vi "EnFlo_Error_Handler.vi"(3 "error in (no error)":errorcluster, 4 "Error Type":string, 5 "Dialog Box (T)":bool=TRUE) -> (0 "Continue":bool, 1 "SMS Message":string, 2 "Email Message":string)   [LabVIEW 2016]
uses:
  Controls/Post_Process.ctl
  <vilib>/Utility/error.llb/DialogType.ctl
  Globals/Meas_global.vi
  Globals/Trav_pos_global.vi
  Globals/Preference_global.vi
  Email_transfer_global.vi
  Globals/Dynamic_call_global.ph.vi
panel:
  out "error out":errorcluster
  in  "Case Constant\n(See Context Help)":bool
  out "Server copy Location":path
  out "Hours Running":dbl format="%.2f"
  out "Error Information":string
  out "Log Files":path[](array[path])
  out "Frequency":i32
  out "Error Analysis":string
  out "Error Types":string[](array[string])
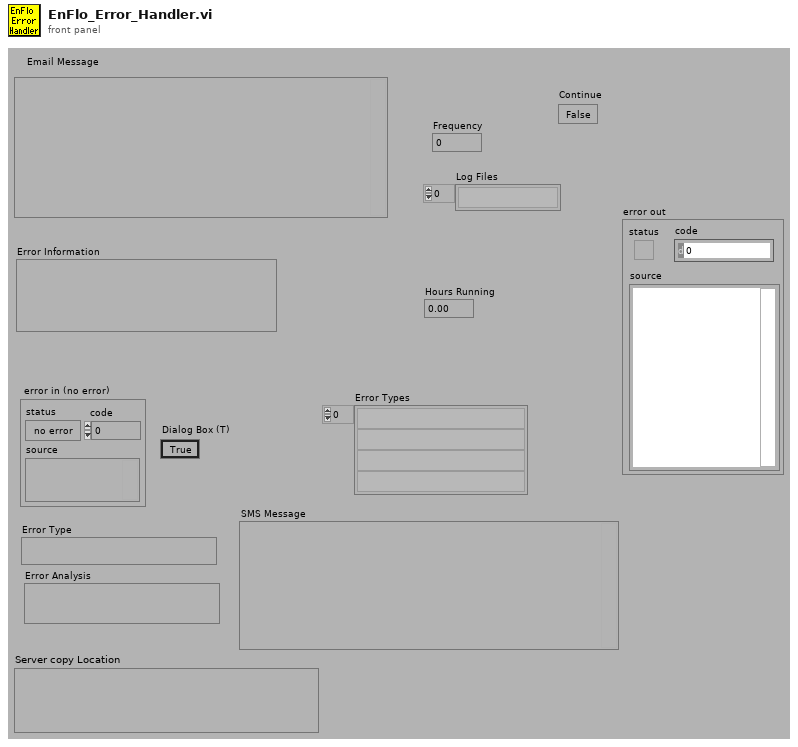
[diagram p1: front panel]
types:
  T1 = typedef "Post_Process.ctl" = enum16{"Take New Data", "Post Process Raw Data File"}
  T2 = cluster{"path":path, "data":string, "binary":bool, "MIME content-type \n(application/octet-stream)":string}[]
  T3 = typedef "DialogType.ctl" = u16
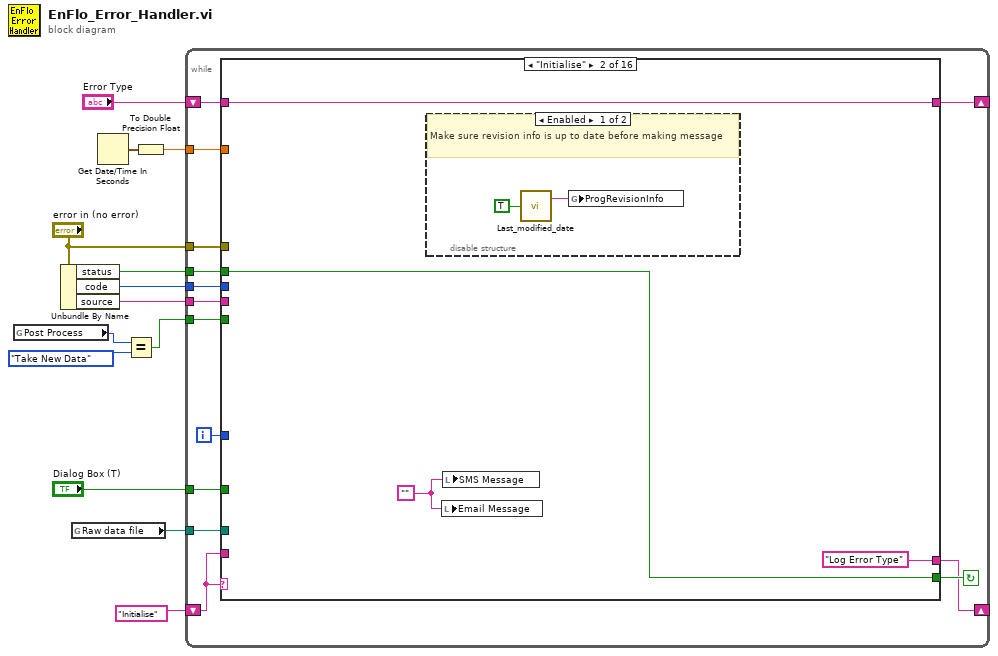
[diagram p0: block diagram]
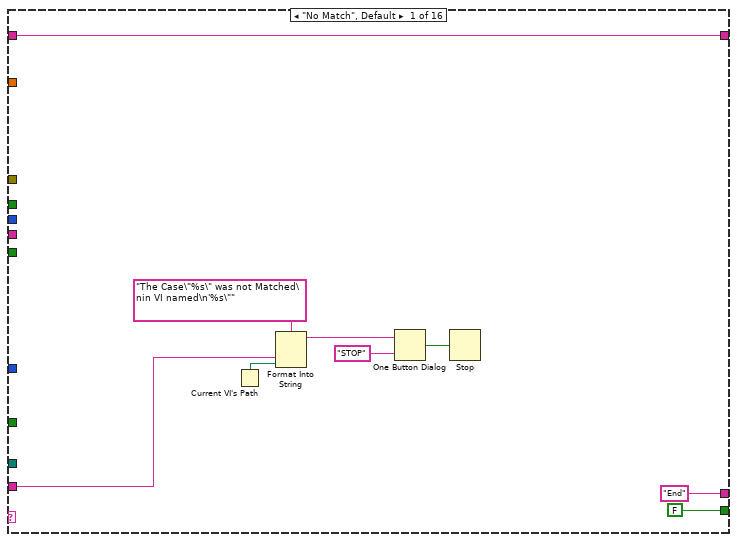
[diagram p2: hidden frame]
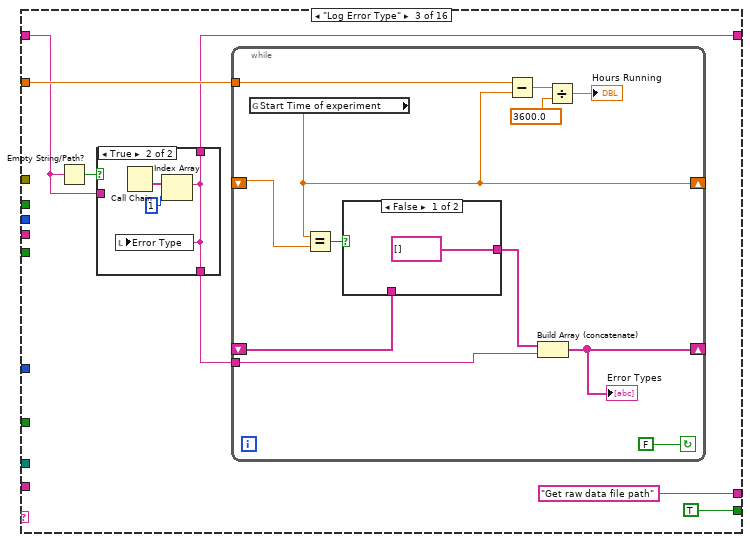
[diagram p4: hidden frame]
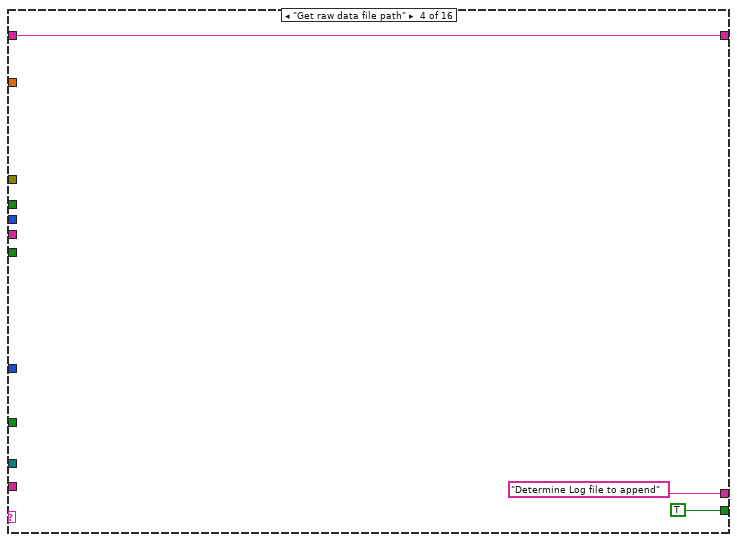
[diagram p7: hidden frame]
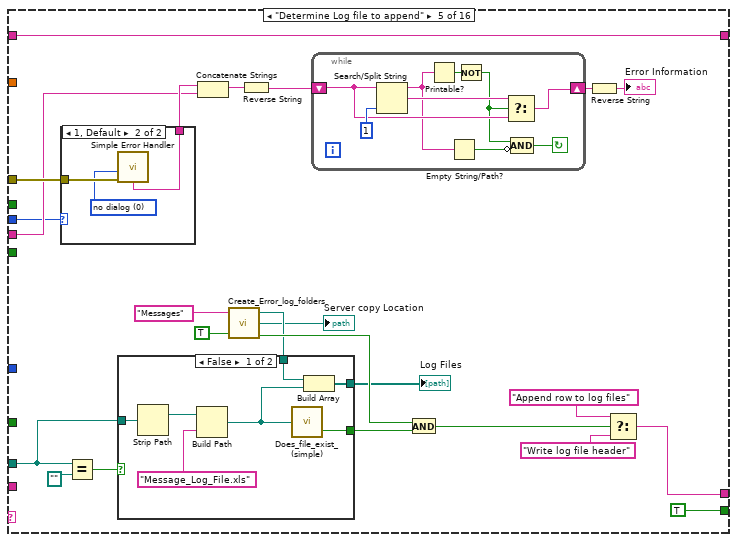
[diagram p8: hidden frame]
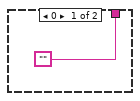
[diagram p9: hidden frame]
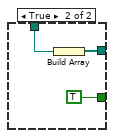
[diagram p10: hidden frame]
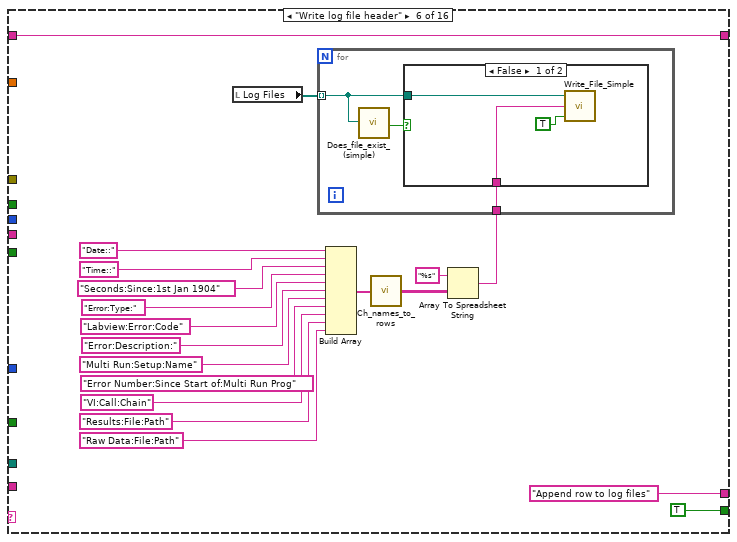
[diagram p11: hidden frame]
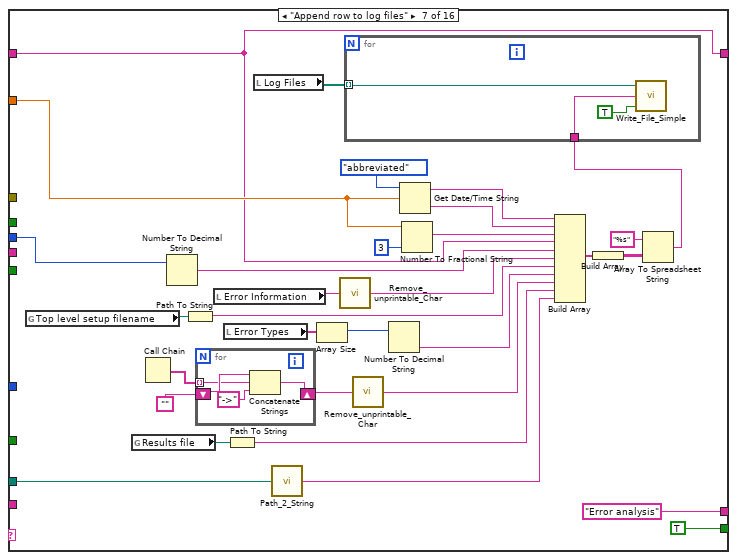
[diagram p13: hidden frame]
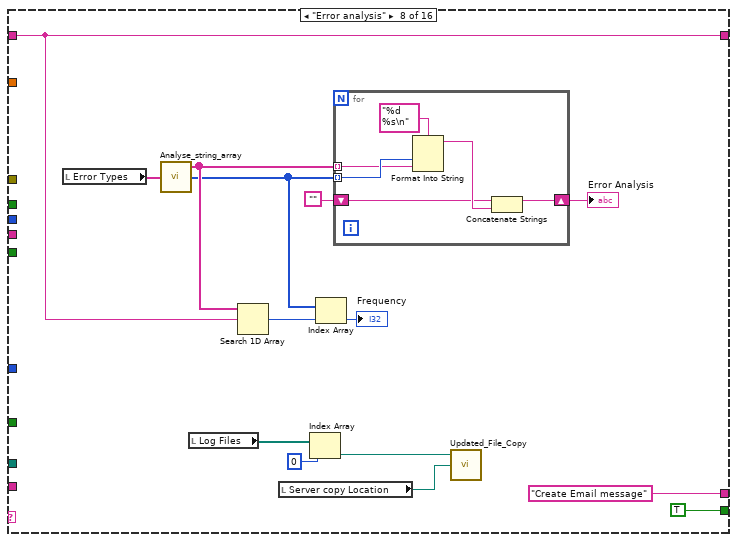
[diagram p14: hidden frame]
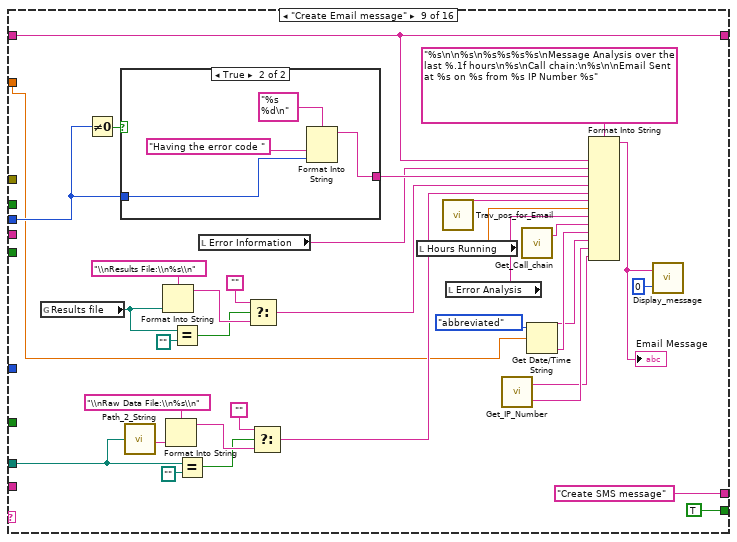
[diagram p15: hidden frame]
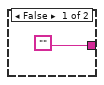
[diagram p16: hidden frame]
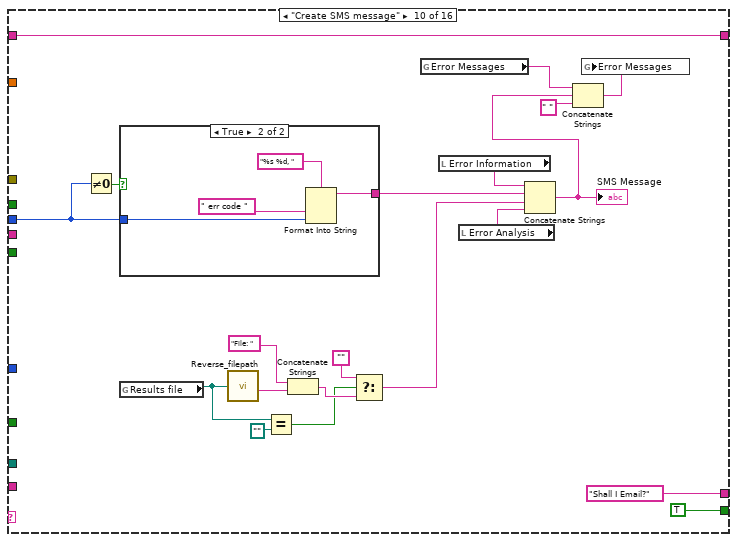
[diagram p17: hidden frame]
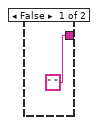
[diagram p18: hidden frame]
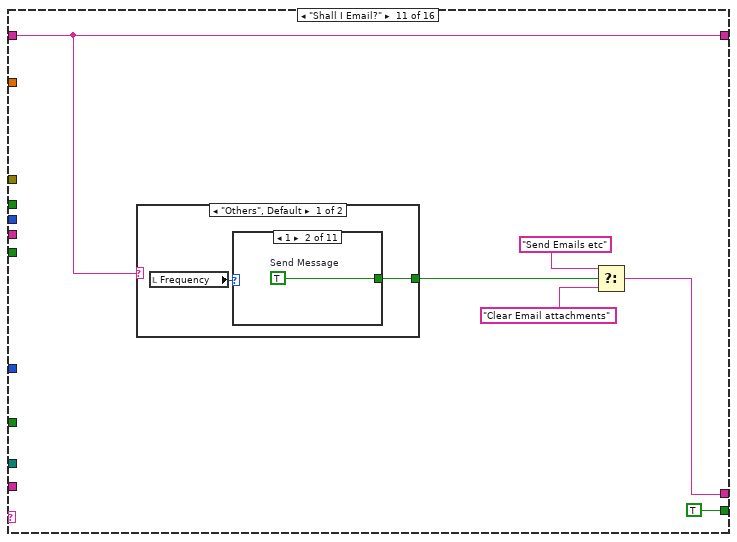
[diagram p19: hidden frame]
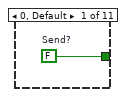
[diagram p20: hidden frame]
diagram:
  n1 = global read "Meas_global.vi" "Post Process"() -> (w6:T1)
  n2 = Unbundle By Name("error in (no error)") -> ("status"=w12:bool, "code"=w11:i32, "source"=w10:string)
  n3 = global read "Meas_global.vi" "Raw data file"() -> (w1:path)
  n4 = Get Date/Time In Seconds() -> (seconds since 1Jan1904=w9:timestamp)
  n5 = Equal?(x=w6, y=Post_Process."Take New Data" ("Post Process")) -> (x = y?=w4:bool)
  n6 = To Double Precision Float(number=w9) -> (double precision float=w13:dbl)
  n7 = while {
    tunnel: w10 -> [w21]
    tunnel: w11 -> [w23]
    tunnel: w12 -> [w24]
    tunnel: w13 -> [w25]
    shift-left: "Initialise" -> [w20]
    shift-right: [w26] -> _
    shift-right: [w18] -> _
    shift-left: "Error Type" -> [w19]
    tunnel: w4 -> [w17]
    tunnel: "Dialog Box (T)" -> [w16]
    tunnel: "error in (no error)" -> [w15]
    tunnel: w1 -> [w14]
    i -> [w22]
    stop <- w27 continue-if-true
    n8 = case shown="\"Initialise\"" w20 {
      tunnel: [FALSE ("Abort") w40 TRUE ("status") TRUE ("status") TRUE ("status") TRUE TRUE TRUE ("status") TRUE ("Abort") TRUE ("status") TRUE ("Abort") TRUE ("Abort") TRUE ("Abort") w337 w348 FALSE ("Abort")] -> w27
      tunnel: ["End" ("f") "Log Error Type" "Get raw data file path" ("f") "Determine Log file to append" ("f") w92 "Append row to log files" ("f") "Error analysis" ("f") "Create Email message" ("f") "Create SMS message" "Shall I Email?" w269 "Clear Email attachments" "Is ADAM scan table running?" ("f") "Show timed error dialog" "Stop" "End"] -> w26
      tunnel: w25 -> [_ _ w46 _ _ _ w148 _ w212 _ _ _ _ _ _ _]
      tunnel: w24 -> [_ w40 _ _ _ _ _ _ _ _ _ _ _ _ _ _]
      tunnel: w23 -> [_ _ _ _ w72 _ w168 _ w234 w259 _ _ _ _ _ _]
      tunnel: w22 -> [_ _ _ _ _ _ _ _ _ _ _ _ _ _ _ _]
      tunnel: w21 -> [_ _ _ _ w74 _ _ _ _ _ _ _ _ _ _ _]
      tunnel: w20 -> [w31 _ _ _ _ _ _ _ _ _ _ _ _ _ _ _]
      tunnel: w19 -> [w28 w37 w44 w68 w79 w118 w145 w186 w206 w241 w271 w289 w335 w339 w346 w352]
      tunnel: [w28 w37 w43 w68 w79 w118 w145 w186 w206 w241 w271 w289 w335 w339 w346 w352] -> w18
      tunnel: w17 -> [_ _ _ _ _ _ _ _ _ _ _ w286 _ _ _ _]
      tunnel: w16 -> [_ _ _ _ _ _ _ _ _ _ _ _ _ w336 _ _]
      tunnel: w15 -> [_ _ _ _ w76 _ _ _ _ _ _ _ _ _ _ _]
      tunnel: w14 -> [_ _ _ _ w71 _ w143 _ w201 _ _ _ _ _ _ _]
      frame "No Match", Default {
        n9 = Current VI's Path() -> (path=w32:path)
        n10 = Format Into String(format string="The Case\"%s\" was not Matched\nin VI named\n'%s\"" ("Format String"), w31, w32) -> (resulting string=w35:string)  [unwired: 2 in, 1 out]
        n11 = One Button Dialog(message=w35, button name ("OK")="STOP") -> (true=w33:bool)
        n12 = Stop(stop? (T)=w33) -> ()
      }
      frame "Initialise" {
        w39 = ""
        n13 = disable-structure shown="Enabled" {
          frame Enabled {
            # "Make sure revision info is up to date before making message"
            n14 = call "Last_modified_date.vi"("Update Now"=TRUE) -> ("RevisionString"=w41:string)  [unwired: 1 out]
            n15 = global write "Meas_global.vi" "ProgRevisionInfo"(w41) -> ()
          }
          frame Disabled {
          }
        }
        n16 = local write "Email Message"(w39) -> ()
        n17 = local write "SMS Message"(w39) -> ()
      }
      frame "Log Error Type" {
        n18 = Empty String/Path?(string/path=w44) -> (empty?=w48:bool)
        n19 = case shown="True" w48 {
          tunnel: [w64 w65] -> w47
          tunnel: w44 -> [w64 _]
          tunnel: [w64 w65] -> w43
          frame False {
          }
          frame True {
            n20 = Call Chain() -> (call chain=w67:string[])
            n21 = Index Array(array=w67, index=1 ("Index")) -> (element=w65:string)
            n22 = local write "Error Type"(w65) -> ()
          }
        }
        n23 = while {
          tunnel: w46 -> [w52]
          shift-left: _ -> [w59]
          shift-right: [w58] -> _
          shift-left: _ -> [w57]
          shift-right: [w55] -> _
          tunnel: w47 -> [w60]
          stop <- FALSE continue-if-true
          n24 = global read "Meas_global.vi" "Start Time of experiment"() -> (w55:dbl)
          n25 = Equal?(x=w55, y=w57) -> (x = y?=w56:bool)
          n26 = case shown="False" w56 {
            tunnel: [string[] [] w63] -> w61
            tunnel: w59 -> [_ w63]
            frame False {
            }
            frame True {
            }
          }
          n27 = Subtract(x=w52, y=w55) -> (x-y=w54:dbl)
          n28 = Build Array (concatenate)(w61, w60) -> (w58:string[])
          "Error Types" <- w58
          n29 = Divide(x=w54, y=3600.0) -> (x/y=→"Hours Running":dbl)
        }
      }
      frame "Get raw data file path" {
      }
      frame "Determine Log file to append" {
        n30 = case shown="1, Default" w72 {
          tunnel: w76 -> [_ w98]
          tunnel: ["" w96] -> w75
          frame 0 {
          }
          frame 1, Default {
            w97 = T3 0 items=["no dialog", "OK message", "continue or stop message", "OK message + warnings", "continue/stop + warnings"] ("type of dialog (OK msg:1)")
            n31 = call <vilib>:"Simple Error Handler.vi"("type of dialog (OK msg:1)"=w97, "error in (no error)"=w98) -> ("message"=w96:string)  [unwired: 7 out]
          }
        }
        n32 = Equal?(x=w71, y=path "") -> (x = y?=w90:bool)
        n33 = Concatenate Strings(w75, w74) -> (w73:string)
        n34 = call "Create_Error_log_folders.vi"("Per Day Log File?"=TRUE, "Log Filename"="Messages" ("Input Element")) -> ("exists?"=w88:bool, "Server copy Location"=→"Server copy Location":path, "Local Log File"=w86:path)  [unwired: 1 in]
        n35 = case shown="False" w90 {
          tunnel: w71 -> [w114 _]
          tunnel: [w111 TRUE ("exists?")] -> w89
          tunnel: w86 -> [w110 w116]
          tunnel: [w108 w115] -> w85
          frame False {
            n36 = Strip Path(path=w114) -> (stripped path=w113:path)  [unwired: 1 out]
            n37 = Build Path(base path=w113, name or relative path="Message_Log_File.xls") -> (appended path=w109:path)
            n38 = call "Does_file_exist_(simple).vi"("Pathname"=w109) -> ("exists?"=w111:bool)
            n39 = Build Array(w110, w109) -> (w108:path[])
          }
          frame True {
            n40 = Build Array(w116) -> (w115:path[])
          }
        }
        "Log Files" <- w85
        n41 = Reverse String(1:w73) -> (0:w84:string)
        n42 = while {
          shift-left: w84 -> [w105]
          shift-right: [w104] -> w83
          stop <- w99 continue-if-true
          n43 = Search/Split String(string=w105, offset (0)=1 ("length")) -> (substring before match=w102:string, match + rest of string=w106:string)  [unwired: 2 out]
          n44 = Printable?(1:w102) -> (0:w103:bool)
          n45 = Empty String/Path?(string/path=w102) -> (empty?=w100:bool)
          n46 = Not(x=w103) -> (.not. x?=w101:bool)
          n47 = Select(t=w106, s=w101, f=w105) -> (s? t:f=w104:string)
          n48 = Compound Arithmetic op=AND(w101, invert w100) -> (w99:bool)
        }
        n49 = And(x=w88, y=w89) -> (x .and. y?=w87:bool)
        n50 = Reverse String(1:w83) -> (0:→"Error Information":string)
        n51 = Select(t="Append row to log files", s=w87, f="Write log file header") -> (s? t:f=w92:string)
      }
      frame "Write log file header" {
        n52 = local read "Log Files"() -> (w122:path[])
        n53 = Build Array("Date::", "Time::", "Seconds:Since:1st Jan 1904", "Error:Type:", "Labview:Error:Code", "Error:Description:", "Multi Run:Setup:Name", "Error Number:Since Start of:Multi Run Prog", "VI:Call:Chain", "Results:File:Path", "Raw Data:File:Path") -> (w121:string[])
        n54 = call "Ch_names_to_rows.vi"("Channel Names"=w121) -> ("3 Row names"=w120:string[][])
        n55 = Array To Spreadsheet String(array=w120, 3:"%s" ("format string")) -> (spreadsheet string=w126:string)  [unwired: 1 out]
        n56 = for {
          tunnel: w126 -> [w139]
          tunnel: w122 -> [w137] mode=indexing
          n57 = call "Does_file_exist_(simple).vi"("Pathname"=w137) -> ("exists?"=w138:bool)
          n58 = case shown="False" w138 {
            tunnel: w139 -> [w141 _]
            tunnel: w137 -> [w140 _]
            frame False {
              n59 = call "Write_File_Simple.vi"("append to file? (new file:F)"=TRUE, "character string"=w141, "file path"=w140) -> ()  [unwired: 2 out]
            }
            frame True {
            }
          }
        }
      }
      frame "Append row to log files" {
        n60 = global read "Trav_pos_global.vi" "Top level setup filename"() -> (w170:path)
        n61 = global read "Meas_global.vi" "Results file"() -> (w153:path)
        n62 = Call Chain() -> (call chain=w158:string[])
        n63 = Number To Decimal String(number=w168) -> (decimal integer string=w167:string)  [unwired: 1 out]
        n64 = Path To String(path=w170) -> (string=w165:string)
        n65 = for {
          shift-right: [w177] -> w157
          shift-left: "" -> [w180]
          tunnel: w158 -> [w179] mode=indexing
          n66 = Concatenate Strings(w180, w179, "->" ("Substring")) -> (w177:string)
        }
        n67 = local read "Error Information"() -> (w150:string)
        n68 = local read "Error Types"() -> (w163:string[])
        n69 = Path To String(path=w153) -> (string=w152:string)
        n70 = local read "Log Files"() -> (w151:path[])
        n71 = call "Path_2_String.vi"("Real Path"=w143) -> ("Path String"=w144:string)
        n72 = Array Size(array=w163) -> (size(s)=w169:i32)
        n73 = call "Remove_unprintable_Char.vi"("Input String"=w150) -> ("Output String"=w166:string)
        n74 = call "Remove_unprintable_Char.vi"("Input String"=w157) -> ("Output String"=w159:string)
        n75 = Number To Decimal String(number=w169) -> (decimal integer string=w164:string)  [unwired: 1 out]
        n76 = Get Date/Time String(date format (0)=enum16{"short", "long", "abbreviated"}."abbreviated", seconds (now)=w148) -> (date string=w172:string, time string=w171:string)  [unwired: 1 out]
        n77 = Number To Fractional String(number=w148, precision (6)=i16 3) -> (F-format string=w147:string)  [unwired: 2 out]
        n78 = Build Array(w172, w171, w147, w145, w167, w166, w165, w164, w159, w152, w144) -> (w154:string[])
        n79 = Build Array(w154) -> (w162:string[][])
        n80 = Array To Spreadsheet String(array=w162, 3:"%s" ("format string")) -> (spreadsheet string=w160:string)  [unwired: 1 out]
        n81 = for {
          tunnel: w160 -> [w175]
          tunnel: w151 -> [w174] mode=indexing
          n82 = call "Write_File_Simple.vi"("append to file? (new file:F)"=TRUE, "character string"=w175, "file path"=w174) -> ()  [unwired: 2 out]
        }
      }
      frame "Error analysis" {
        n83 = local read "Error Types"() -> (w189:string[])
        n84 = call "Analyse_string_array.vi"("String array"=w189) -> ("Unique strings"=w193:string[], "Frequency"=w192:i32[])  [unwired: 1 out]
        n85 = local read "Log Files"() -> (w184:path[])
        n86 = Search 1D Array(1D array=w193, element=w186) -> (index of element=w194:i32)  [unwired: 1 out]
        n87 = local read "Server copy Location"() -> (w181:path)
        n88 = Index Array(array=w184, index=0) -> (element=w182:path)
        n89 = Index Array(array=w192, index=w194) -> (element=→"Frequency":i32)
        n90 = for {
          tunnel: w193 -> [w198] mode=indexing
          tunnel: w192 -> [w199] mode=indexing
          shift-right: [w195] -> w190
          shift-left: "" -> [w196]
          n91 = Format Into String(format string="%d %s\n" ("Format String"), w199, w198) -> (resulting string=w197:string)  [unwired: 2 in, 1 out]
          n92 = Concatenate Strings(w196, w197) -> (w195:string)
        }
        "Error Analysis" <- w190
        n93 = call "Updated_File_Copy.vi"("Target Path"=w181, "Source Path"=w182) -> ()  [unwired: 2 out]
      }
      frame "Create Email message" {
        n94 = global read "Meas_global.vi" "Results file"() -> (w219:path)
        n95 = Not Equal To 0?(x=w234) -> (x != 0?=w235:bool)
        n96 = case shown="True" w235 {
          tunnel: w234 -> [_ w239]
          tunnel: ["" w237] -> w233
          frame False {
          }
          frame True {
            n97 = Format Into String(format string="%s %d\n" ("Format String"), "Having the error code ", w239) -> (resulting string=w237:string)  [unwired: 2 in, 1 out]
          }
        }
        n98 = call "Path_2_String.vi"("Real Path"=w201) -> ("Path String"=w204:string)
        n99 = Format Into String(format string="\\nResults File:\\n%s\\n" ("Format String"), w219) -> (resulting string=w225:string)  [unwired: 2 in, 1 out]
        n100 = Format Into String(format string="\\nRaw Data File:\\n%s\\n" ("Format String"), w204) -> (resulting string=w223:string)  [unwired: 2 in, 1 out]
        n101 = Equal?(x=w219, y=path "") -> (x = y?=w218:bool)
        n102 = Equal?(x=w201, y=path "") -> (x = y?=w220:bool)
        n103 = local read "Error Information"() -> (w217:string)
        n104 = Select(t="", s=w218, f=w225) -> (s? t:f=w228:string)
        n105 = Select(t="", s=w220, f=w223) -> (s? t:f=w227:string)
        n106 = local read "Hours Running"() -> (w215:dbl)
        n107 = call "Trav_pos_for_Email.vi"() -> ("String"=w216:string)
        n108 = local read "Error Analysis"() -> (w214:string)
        n109 = call "Get_IP_Number.vi"() -> ("Computer Name"=w203:string, "IP Number"=w202:string)
        n110 = call "Get_Call_chain.vi"() -> ("Output String"=w213:string)  [unwired: 1 in, 1 out]
        n111 = Get Date/Time String(date format (0)=enum16{"short", "long", "abbreviated"}."abbreviated", seconds (now)=w212) -> (date string=w208:string, time string=w210:string)  [unwired: 1 out]
        n112 = Format Into String(format string="%s\n\n%s\n%s%s%s%s\nMessage Analysis over the last %.1f hours\n%s\nCall chain:\n%s\n\nEmail Sent at %s on %s from %s IP Number %s" ("Format String"), w206, w217, w233, w228, w227, w216, w215, w214, w213, w210, w208, w203, w202) -> (resulting string=w209:string)  [unwired: 2 in, 1 out]
        "Email Message" <- w209
        n113 = call "Display_message.vi"("Time to display message"=u32 0, "Message"=w209) -> ()  [unwired: 2 out]
      }
      frame "Create SMS message" {
        n114 = Not Equal To 0?(x=w259) -> (x != 0?=w260:bool)
        n115 = case shown="True" w260 {
          tunnel: w259 -> [_ w264]
          tunnel: [" " w262] -> w258
          frame False {
          }
          frame True {
            n116 = Format Into String(format string="%s %d, " ("Format String"), " err code ", w264) -> (resulting string=w262:string)  [unwired: 2 in, 1 out]
          }
        }
        n117 = global read "Meas_global.vi" "Results file"() -> (w245:path)
        n118 = call "Reverse_filepath.vi"("Filename"=w245) -> ("Reversed Filepath"=w252:string)
        n119 = Equal?(x=w245, y=path "") -> (x = y?=w244:bool)
        n120 = Concatenate Strings("File: ", w252) -> (w250:string)
        n121 = Select(t="", s=w244, f=w250) -> (s? t:f=w248:string)
        n122 = global read "Meas_global.vi" "Error Messages"() -> (w255:string)
        n123 = local read "Error Information"() -> (w243:string)
        n124 = local read "Error Analysis"() -> (w247:string)
        n125 = Concatenate Strings(w243, w258, w248, w247) -> (w253:string)
        "SMS Message" <- w253
        n126 = Concatenate Strings(w255, w253, " ") -> (w254:string)
        n127 = global write "Meas_global.vi" "Error Messages"(w254) -> ()
      }
      frame "Shall I Email?" {
        n128 = case shown="\"Others\", Default" w271 {
          tunnel: [w272 TRUE ("Send Message")] -> w270
          frame "Others", Default {
            n129 = local read "Frequency"() -> (w273:i32)
            n130 = case shown="1" w273 {
              tunnel: [w274 w275 w276 w277 TRUE TRUE TRUE TRUE TRUE TRUE w284] -> w272
              frame 0, Default {
                w274 = FALSE  # Send?
              }
              frame 1 {
                w275 = TRUE  # Send Message
              }
              frame 2 {
                w276 = TRUE  # Send Message
              }
              frame 5 {
                w277 = TRUE  # Send Message
              }
              frame 10 {
              }
              frame 20 {
              }
              frame 50 {
              }
              frame 100 {
              }
              frame 200 {
              }
              frame 500 {
              }
              frame 1000 {
                w284 = TRUE  # Send Message
              }
            }
          }
          frame "Message" {
          }
        }
        n131 = Select(t="Send Emails etc", s=w270, f="Clear Email attachments") -> (s? t:f=w269:string)
      }
      frame "Send Emails etc" {
        n132 = global read "Preference_global.vi" "LabVIEW Administrators"() -> (w287:string[])
        n133 = case shown="True" w286 {
          tunnel: w289 -> [_ w292]
          tunnel: w287 -> [_ w291]
          frame False {
          }
          frame True {
            n134 = stacked-sequence {
              tunnel: w292 -> [_ w297 _ _ w319]
              tunnel: w291 -> [w294 _ w311 _ _]
              frame #0 {
                n135 = global read "Meas_global.vi" "People to Email"() -> (w293:string[])
                n136 = global read "Email_transfer_global.vi" "recipients"() -> (w295:string[])
                n137 = Build Array (concatenate)(w295, w294, w293) -> (w296:string[])
                n138 = global write "Email_transfer_global.vi" "recipients"(w296) -> ()
              }
              frame #1 {
                n139 = global write "Email_transfer_global.vi" "subject ([No Subject])"(w297) -> ()
              }
              frame #2 {
                n140 = local read "Email Message"() -> (w298:string)
                n141 = Concatenate Strings(w298, "\nThis email has been generated  automatically by LabVIEW. If you need help with understanding the email, or want to be removed from the mailing list please contact:\n") -> (w309:string)
                n142 = Concatenate Strings(" or ", "\n") -> (w305:string)
                n143 = for {
                  shift-right: [w313] -> w308
                  shift-left: w309 -> [w315]
                  tunnel: w311 -> [w314] mode=indexing
                  tunnel: w305 -> [w312]
                  n144 = Concatenate Strings(w315, w314, w312) -> (w313:string)
                }
                n145 = String Length(string=w305) -> (length=w303:i32)
                n146 = String Length(string=w308) -> (length=w304:i32)
                n147 = Subtract(x=w304, y=w303) -> (x-y=w302:i32)
                n148 = String Subset(string=w308, length (rest)=w302) -> (substring=w301:string)  [unwired: 1 out]
                n149 = Concatenate Strings(w301, "\n") -> (w299:string)
                n150 = global write "Email_transfer_global.vi" "message"(w299) -> ()
              }
              frame #3 {
                n151 = call "Launch_Async_Email.vi"() -> ("error out"=→"error out":errorcluster)  [unwired: 2 out]
              }
              frame #4 {
                n152 = local read "Frequency"() -> (w317:i32)
                n153 = case shown="\"Warning\"" w319 {
                  tunnel: [TRUE FALSE w327 FALSE] -> w321
                  tunnel: w317 -> [_ _ w329 _]
                  frame "No Match", Default {
                  }
                  frame "Pulse Width Error" {
                  }
                  frame "LDA Invalid Bursts" {
                    n154 = Greater?(x=w329, y=4) -> (0:w327:bool)
                  }
                  frame "Warning" {
                  }
                }
                n155 = local read "SMS Message"() -> (w320:string)
                n156 = global read "Meas_global.vi" "People to Email"() -> (w318:string[])
                n157 = case shown="True" w321 {
                  tunnel: w320 -> [_ w324]
                  tunnel: w318 -> [_ w323]
                  tunnel: w319 -> [_ w322]
                  frame False {
                  }
                  frame True {
                    n158 = call "SMS_to_mobile.vi"("SMS address"=w323, "Subject"=w322, "Message"=w324) -> ()  [unwired: 3 out]
                  }
                }
              }
            }
          }
        }
      }
      frame "Clear Email attachments" {
        n159 = global write "Email_transfer_global.vi" "attachments"(T2 [] ("attachments")) -> ()
        n160 = global write "Email_transfer_global.vi" "recipients"(string[] [] ("recipients")) -> ()
      }
      frame "Is ADAM scan table running?" {
        n161 = Open VI Reference(vi path="ADAM_scan_table.vi") -> (vi reference=w343:refnum<vi>, error out=w342:errorcluster)  [unwired: 1 in, 4 out]
        n162 = Unbundle By Name(w342) -> ("status"=w338:bool)
        n163 = case shown="False" w338 {
          tunnel: w342 -> [w345 _]
          tunnel: w343 -> [w344 _]
          frame False {
            n164 = Close Reference(reference=w344, error in (no error)=w345) -> ()  [unwired: 1 out]
          }
          frame True {
          }
        }
        n165 = Compound Arithmetic op=AND(w338, w336) -> (w337:bool)
      }
      frame "Show timed error dialog" {
        n166 = local read "Email Message"() -> (w350:string)
        n167 = call "Timed_Error_dialog.vi"("Message"=w350, "Seconds to wait"=60.0) -> ("Ignore"=→"Continue":bool, "Abort"=w348:bool)
      }
      frame "Stop" {
        n168 = stacked-sequence {
          seq-local: [_ w362 _ _ _] -> [_ _ w376 _ _]
          frame #0 {
            n169 = call "Program_Active_Aborting.vi"() -> ()  [unwired: 6 out]
          }
          frame #1 {
            n170 = Build Array("Edit_BSA_setup.vi", "Measurement_input_panel.vi", "Input_Value_Dialog.vi", "Input_String_Dialog.vi", "Calibration_user_input.vi", "Input_Traverse_position.vi", "User_Metadata.vi", "Preference_Panel.vi", "Traverse_Space.vi", "Enter_Temp_Press.vi", "EnFlo_Tunnel_Setup.vi", "Gas_Setup.vi", "Correlation_Display.vi", "Serial_Setup.vi", "Port_Names.vi", "Select_Strings.vi", "Edit_Template_File.vi", "Select_a_Channel.vi", "Output_file_Panel.vi", "Enter_LDA_Setup.vi") -> (w362:string[])
          }
          frame #2 {
            n171 = for {
              tunnel: w376 -> [w377] mode=indexing
              n172 = Open VI Reference(vi path=w377) -> (vi reference=w382:refnum<vi>, error out=w381:errorcluster)  [unwired: 1 in, 4 out]
              n173 = property class="VI"(reference=w382, error in=w381, "Front Panel Window:Open"=FALSE) -> (reference out=w380:refnum<vi>, error out=w379:errorcluster)
              n174 = Close Reference(reference=w380, error in (no error)=w379) -> ()  [unwired: 1 out]
            }
          }
          frame #3 {
            n175 = case shown="True" "Case Constant\n(See Context Help)" {
              frame False {
              }
              frame True {
                # "Cased out 4/7/07 because it hung code"
                n176 = global write "Dynamic_call_global.ph.vi" "EnFlo Hub running?"(FALSE ("EnFlo Hub running?")) -> ()
              }
            }
          }
          frame #4 {
            n177 = Stop(stop? (T)=TRUE) -> ()
          }
        }
      }
    }
  }
